vi "Timeout.vi"(8 "error in":errorcluster, 11 "Main Data Buffer In":T2) -> (0 "error out":errorcluster, 1 "On-Line":bool, 2 "HSMS State":T1=enum."Stop", 3 "Main Data Buffer Out":T2, 5 "Version":string)   [LabVIEW 2020, in "SECS Bridge.lvlib"]
uses:
  SECS Bridge.lvlib
  Main Data Buffer.ctl
  SECS Communication/HSMS Class/HSMS Class.lvclass
  SECS Communication/SECS Data Class/SECS Data Class.lvclass
  SECS Scenarios/Scenarios Class/Scenarios Class.lvclass
  SECS Communication/HSMS Class/HSMS State.ctl
  SECS Communication/HSMS Class/HSMS Class.lvclass/HSMS Class.ctl
  7d990879-b174-4d9d-8932-9c39beb10743.vi
  240646f7-56f9-43de-8349-65f83add290a.vi
  SECS Communication/HSMS Class/Read HSMS State.vi
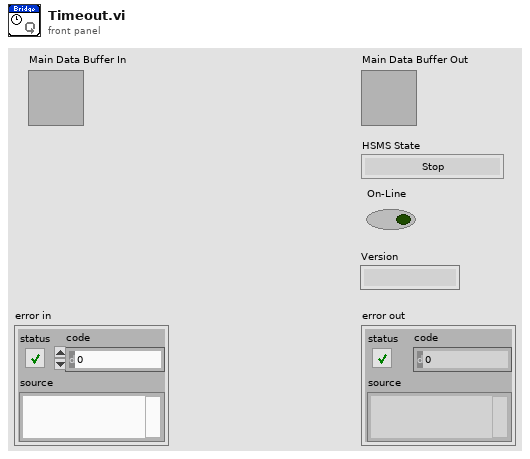
[diagram p1: front panel]
types:
  T1 = typedef "SECS Communication.lvlib/HSMS Class.lvclass/HSMS State.ctl" = enum16{"[TCP/IP]Not Connect", "[HSMS]Not Selected", "[HSMS]Selected", "Stop"}
  T2 = typedef "SECS Bridge.lvlib/Main Data Buffer.ctl" = cluster{"HSMS Class":refnum<class "HSMS Class.lvclass">, "SECS Data Class":refnum<class "SECS Data Class.lvclass">, "Scenarios Class":refnum<class "Scenarios Class.lvclass">, "VI Refnum":refnum<vi>, "Ctl Refnum Map":map{string, refnum<vi>}, "Timeout":i32, "Notifier Data":string[], "Event Refnum":refnum<event-registration>}
  T3 = cluster{"Major":u16, "Minor":u16, "Fix":u16, "Build":u16}
  T4 = typedef "SECS Bridge.lvlib/Broadcast Refnum.ctl" = cluster{"Nottifier Data User Event":refnum<user-event>, "HSMS State User Event":refnum<user-event>, "On-Line User Event":refnum<user-event>}
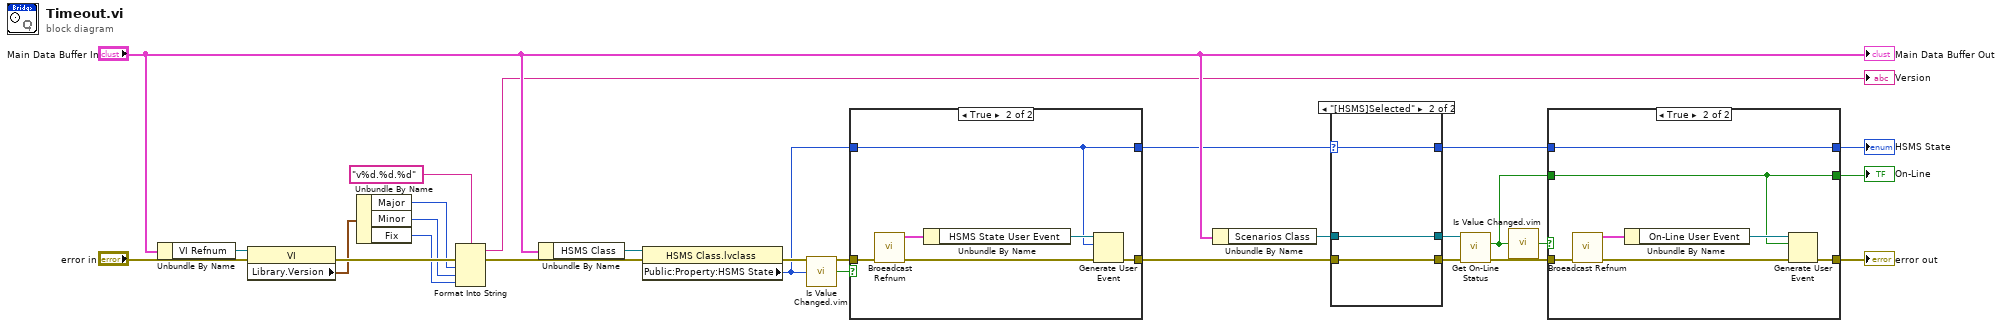
[diagram p0: block diagram]
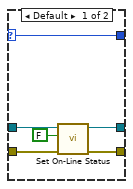
[diagram p4: hidden frame]
diagram:
  n1 = Unbundle By Name("Main Data Buffer In") -> ("VI Refnum"=w24:refnum<vi>)
  n2 = property class="VI"(reference=w24, error in="error in") -> (error out=w23:errorcluster, "Library.Version"=w21:T3)  [unwired: 1 out]
  n3 = Unbundle By Name(w21) -> ("Major"=w18:u16, "Minor"=w19:u16, "Fix"=w20:u16)
  n4 = Format Into String(format string="v%d.%d.%d", error in=w23, w18, w19, w20) -> (resulting string=→"Version":string, error out=w22:errorcluster)  [unwired: 1 in]
  n5 = Unbundle By Name("Main Data Buffer In") -> ("HSMS Class"=w27:refnum<class "HSMS Class.lvclass">)
  n6 = property class="HSMS Class.lvclass"(reference=w27, error in=w22) -> (error out=w11:errorcluster, "Public:Property:HSMS State"=w10:T1)  [unwired: 1 out]
  n7 = call "Is Value Changed.vim"("value"=w10) -> ("changed or first call?"=w12:bool)
  n8 = case shown="True" w12 {
    tunnel: w11 -> [w28 w32]
    tunnel: w10 -> [w29 w31]
    tunnel: [w29 w31] -> w9
    tunnel: [w28 w30] -> w8
    frame False {
    }
    frame True {
      n9 = call "Broeadcast Refnum.vi"("error in"=w32) -> ("error out"=w35:errorcluster, "Broadcast Refnum"=w33:T4)  [unwired: 9 in]
      n10 = Unbundle By Name(w33) -> ("HSMS State User Event"=w34:refnum<user-event>)
      n11 = Generate User Event(user event=w34, event data cluster=w31, error in=w35) -> (error out=w30:errorcluster)  [unwired: 1 in, 1 out]
    }
  }
  n12 = Unbundle By Name("Main Data Buffer In") -> ("Scenarios Class"=w14:refnum<class "Scenarios Class.lvclass">)
  n13 = case shown="\"[HSMS]Selected\"" w9 {
    selector: w9 -> [w39 w44]
    tunnel: w8 -> [w41 w42]
    tunnel: [w39 w44] -> w6
    tunnel: [w38 w42] -> w15
    tunnel: w14 -> [w40 w43]
    tunnel: [w36 w43] -> w13
    frame Default {
      n14 = call "Set On-Line Status.vi"("error in (no error)"=w41, "On-Line"=FALSE, "Scenarios Class in"=w40) -> ("error out"=w38:errorcluster, "Scenarios Class out"=w36:refnum<class "Scenarios Class.lvclass">)  [unwired: 7 in]
    }
    frame "[HSMS]Selected" {
    }
  }
  n15 = call "Get On-Line Status.vi"("error in (no error)"=w15, "Scenarios Class in"=w13) -> ("error out"=w7:errorcluster, "On-Line"=w4:bool)  [unwired: 7 in, 1 out]
  n16 = call "Is Value Changed.vim"("value"=w4) -> ("changed or first call?"=w3:bool)
  n17 = case shown="True" w3 {
    tunnel: w7 -> [w46 w51]
    tunnel: w6 -> [w47 w50]
    tunnel: [w47 w50] -> w2
    tunnel: [w46 w49] -> w1
    tunnel: w4 -> [w45 w48]
    tunnel: [w45 w48] -> w5
    frame False {
    }
    frame True {
      n18 = call "Broeadcast Refnum.vi"("error in"=w51) -> ("error out"=w54:errorcluster, "Broadcast Refnum"=w52:T4)  [unwired: 9 in]
      n19 = Unbundle By Name(w52) -> ("On-Line User Event"=w53:refnum<user-event>)
      n20 = Generate User Event(user event=w53, event data cluster=w48, error in=w54) -> (error out=w49:errorcluster)  [unwired: 1 in, 1 out]
    }
  }
  "error out" <- w1
  "HSMS State" <- w2
  "On-Line" <- w5
  "Main Data Buffer Out" <- "Main Data Buffer In"
